vi "Write menu reference.vi"(8 "error in (no error)":errorcluster, 10 "menu reference":refnum<k9>, 11 "Waveform_Task in":refnum<class "Waveform_Task.lvclass">) -> (0 "error out":errorcluster, 3 "Waveform_Task out":refnum<class "Waveform_Task.lvclass">)   [LabVIEW 2025, in "Waveform_Task.lvlib" / "Waveform_Task.lvclass"]
uses:
  Waveform_Task.lvclass
  Waveform_Task.lvclass/Waveform_Task.ctl
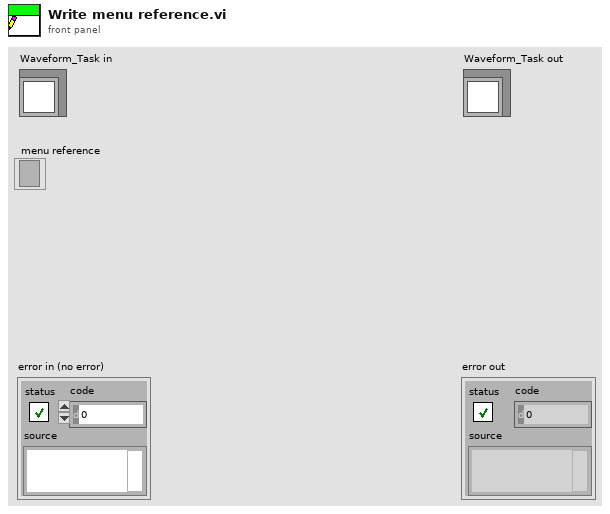
[diagram p1: front panel]
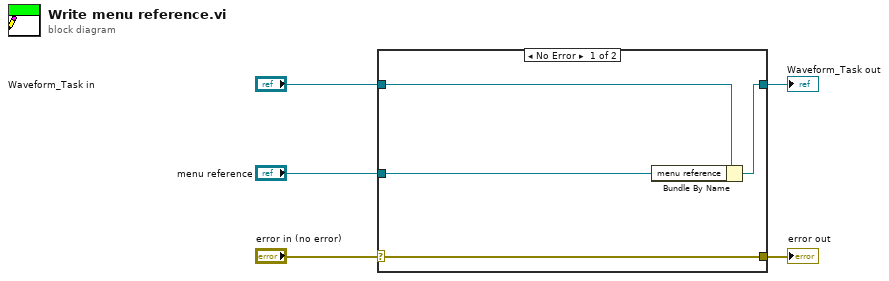
[diagram p0: block diagram]
diagram:
  n1 = case shown="No Error" "error in (no error)" {
    selector: "error in (no error)" -> [w9 w10]
    tunnel: [w9 w10] -> w4
    tunnel: [w7 w11] -> w2
    tunnel: "Waveform_Task in" -> [w8 w11]
    tunnel: "menu reference" -> [w6 _]
    frame No Error {
      n2 = Bundle By Name(cluster=w8, "menu reference"=w6) -> (w7:refnum<class "Waveform_Task.lvclass">)
    }
    frame Error {
    }
  }
  "error out" <- w4
  "Waveform_Task out" <- w2
